vi "Lookup Indicator Type.vi"(10 "error in (no error)":errorcluster, 11 "Indicator Type":string) -> (2 "error out":errorcluster, 3 "Indicator":refnum<class "Indicator.lvclass">)   [LabVIEW 2020, in "VolatusGUI.lvlib"]
uses:
  VolatusGUI.lvlib
  Indicator/Indicator.lvclass
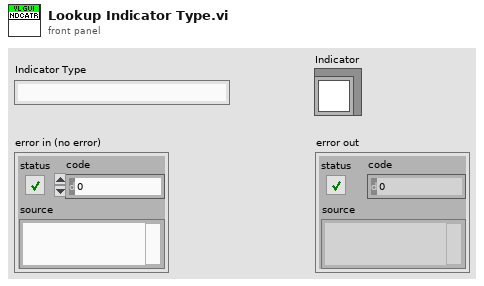
[diagram p1: front panel]
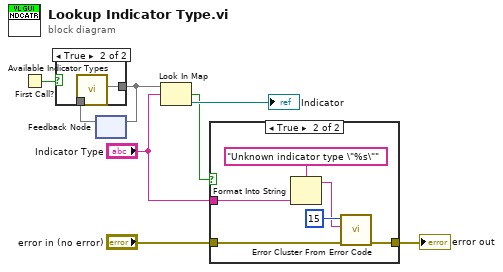
[diagram p0: block diagram]
diagram:
  n1 = First Call?() -> (First Call?: T/F=w8:bool)
  n2 = feedback #1() -> (w7:map{string, refnum<class "Indicator.lvclass">})  [unwired: 1 in]
  n3 = case shown="True" w8 {
    tunnel: [w9 w10] -> w6
    tunnel: w7 -> [w9 _]
    frame False {
    }
    frame True {
      n4 = call "Available Indicator Types.vi"() -> ("Indicator Types"=w10:map{string, refnum<class "Indicator.lvclass">})  [unwired: 11 in]
    }
  }
  n5 = feedback-in #1(w6) -> ()
  n6 = Look In Map(map=w6, key="Indicator Type") -> (key not found?=w4:bool, value=→"Indicator":refnum<class "Indicator.lvclass">)  [unwired: 1 in]
  n7 = case shown="True" w4 {
    tunnel: "Indicator Type" -> [_ w14]
    tunnel: "error in (no error)" -> [w11 w13]
    tunnel: [w11 w12] -> w1
    frame False {
    }
    frame True {
      n8 = Format Into String(format string="Unknown indicator type \"%s\"", w14) -> (resulting string=w16:string)  [unwired: 2 in, 1 out]
      n9 = call <vilib>:"Error Cluster From Error Code.vi"("error in (no error)"=w13, "error message (\"\")"=w16, "error code (0)"=15) -> ("error out"=w12:errorcluster)  [unwired: 6 in]
    }
  }
  "error out" <- w1
